vi "FrequenzPegelKorrigieren.vi"(9 "gemessenerPegel":dbl[](array[numeric])=[111.51644632809406, 119.57867726956083, 106.23008269385458], 10 "SollPegel":dbl=94.0, 11 "Frequency List":T1(array[cluster])=[{"frequency [Hz]"=10.0, "amplitude [V]"=0.1}, {"frequency [Hz]"=100.0, "amplitude [V]"=0.1}, {"frequency [Hz]"=1000.0, "amplitude [V]"=0.1}]) -> (3 "korrigierte Frequenzliste":T1(array[cluster]))   [LabVIEW 2018]
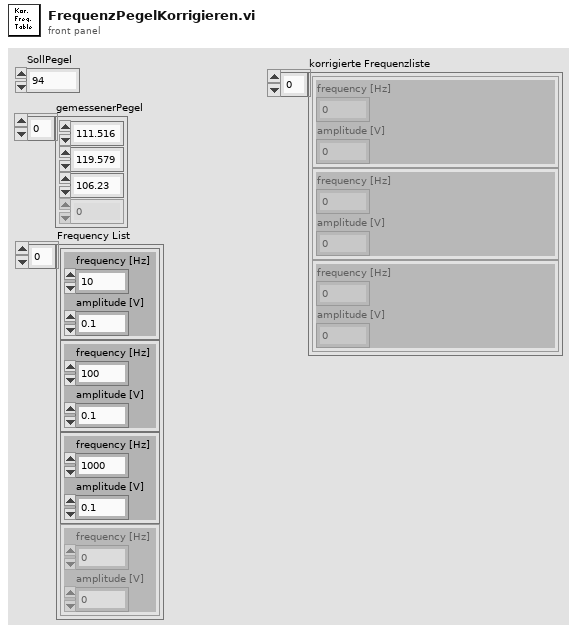
[diagram p1: front panel]
types:
  T1 = cluster{"frequency [Hz]":dbl, "amplitude [V]":dbl}[]
  T2 = cluster{"frequency [Hz]":dbl, "amplitude [V]":dbl}
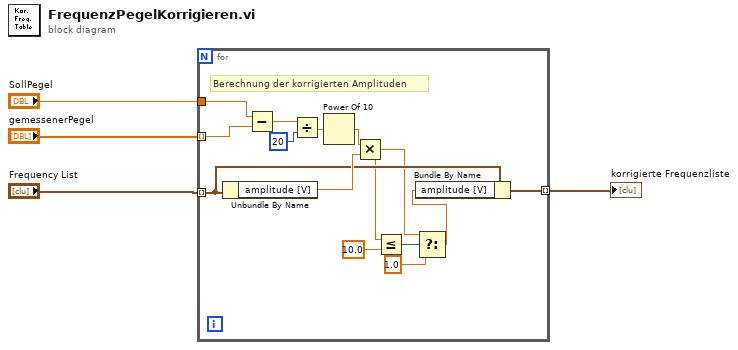
[diagram p0: block diagram]
diagram:
  n1 = for {
    tunnel: "gemessenerPegel" -> [w15] mode=indexing
    tunnel: "SollPegel" -> [w18]
    tunnel: "Frequency List" -> [w10] mode=indexing
    tunnel: [w14] -> w1 mode=indexing
    # "Berechnung der korrigierten Amplituden"
    n2 = Unbundle By Name(w10) -> ("amplitude [V]"=w11:dbl)
    n3 = Subtract(x=w18, y=w15) -> (x-y=w17:dbl)
    n4 = Divide(x=w17, y=20) -> (x/y=w13:dbl)
    n5 = Power Of 10(x=w13) -> (10^x=w12:dbl)
    n6 = Multiply(x=w12, y=w11) -> (x*y=w6:dbl)
    n7 = Less Or Equal?(x=w6, y=10.0) -> (x <= y?=w9:bool)
    n8 = Select(t=w6, s=w9, f=1.0) -> (s? t:f=w8:dbl)
    n9 = Bundle By Name(cluster=w10, "amplitude [V]"=w8) -> (w14:T2)
  }
  "korrigierte Frequenzliste" <- w1
